vi "Sumador.vi"() -> ()   [LabVIEW 2018]
panel:
  out "Suma 2":i32
  out "Suma 1":i32
  in  "stop":bool
  in  "Push 2":bool
  in  "Push 1":bool
  # "Suma sin supresor de rebote"
  # "Suma con supresor de rebote"
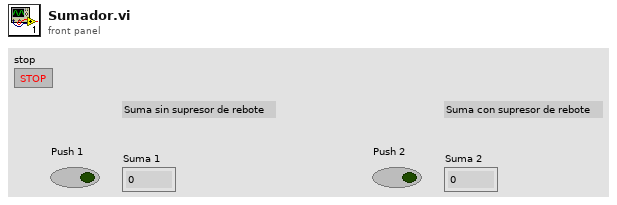
[diagram p1: front panel]
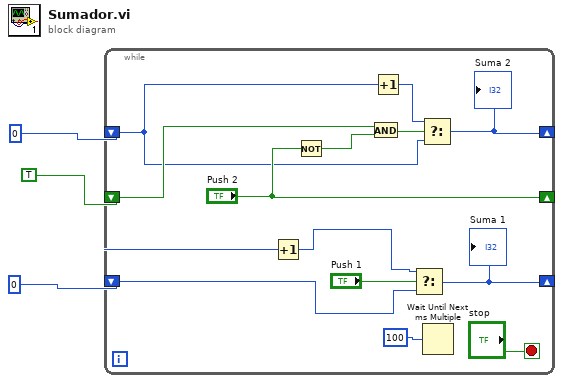
[diagram p0: block diagram]
diagram:
  n1 = while {
    shift-right: [w14] -> _
    shift-left: 0 -> [w4]
    shift-right: ["Push 2"] -> _
    shift-left: TRUE -> [w10]
    shift-right: [w11] -> _
    shift-left: 0 -> [w7]
    stop <- "stop" stop-if-true
    n2 = Increment(x=w4) -> (x+1=w5:i32)
    n3 = Not(x="Push 2") -> (.not. x?=w13:bool)
    n4 = And(x=w10, y=w13) -> (x .and. y?=w12:bool)
    n5 = Increment(x=w7) -> (x+1=w8:i32)
    n6 = Select(t=w5, s="Push 1", f=w4) -> (s? t:f=w14:i32)
    "Suma 1" <- w14
    n7 = Select(t=w8, s=w12, f=w7) -> (s? t:f=w11:i32)
    "Suma 2" <- w11
    n8 = Wait Until Next ms Multiple(millisecond multiple=u32 100) -> ()  [unwired: 1 out]
  }
